vi "add_object.vi"(6 "wait for reply (T)":bool=TRUE, 8 "error in":errorcluster, 9 "object_name":string, 10 "vi_reference":i32) -> (0 "error out":errorcluster, 1 "timed out?":bool, 2 "result":string, 3 "object_id":i32)   [LabVIEW 2025, in "Scripting Server.lvlib"]
doc: "Adds an object to the block diagram or frontpanel of the referenced vi. Get a VI reference from \"New VI\".\nAllowed object names are:\n.NET Container\n.NET Refnum\n2D Picture\n3D Picture\nAbsolute Value\nAccept TLS\nAccess Rights\nActiveX Container\nAdd\nAdd (with error terminals)\nAdd Array Elements\nAdd Entropy\nAdd Private Key To TLS Configuration\nAdd Trusted Certificate To TLS Configuration\nAgitator\nAllSpoll\nAlways Copy\nAnd\nAnd Array Elements\nAppend True/False String\nApplication Refnum\nArray (block diagram constant)\nArray (classic)\nArray (modern)\nArray Interface Control\nArray Max & Min\nArray of Strings to Path\nArray Size\nArray Subset\nArray To Cluster\nArray To Spreadsheet String\nArrayMemInfo\nAssert Structural Type Match\nAssert Structural Type Mismatch\nAtmospheric Tank (classic)\nAtmospheric Tank (modern)\nAutomation Close\nAutomation Open\nAutomation Refnum\nAvogadro Constant (1/mol)\nBase 10 Logarithm Of e\nBin #1\nBin #2\nBitpack to Array\nBluetooth Close Connection\nBluetooth Create Listener\nBluetooth Discover\nBluetooth Network Connection Refnum\nBluetooth Open Connection\nBluetooth Read\nBluetooth Wait On Listener\nBluetooth Write\nBoolean Array To Number\nBoolean To (0,1)\nBuild Array\nBuild Cluster Array\nBuild Map\nBuild Matrix\nBuild Path\nBuild Set\nBuild Waveform\nBundle\nBundle By Name\nByte Array To String\nByte Array To UTF-8 String\nByte Stream File Refnum\nCall By Reference\nCall Chain\nCall Library Function Node\nCall MATLAB Function\nCall Parent Class Method\nCAN Channel (block diagram constant)\nCAN Channel (classic)\nCAN Channel (modern)\nCAN Channel (system)\nCAN Interface (block diagram constant)\nCAN Interface (classic)\nCAN Interface (modern)\nCAN Interface (system)\nCAN Task (block diagram constant)\nCAN Task (classic)\nCAN Task (modern)\nCAN Task (system)\nCancel Button (modern)\nCancel Button (system)\nCancel Notification\nCarriage Return Constant\nCase Structure\nCast Unit Bases\nCheck Valve\nCheckbox (classic)\nCheckBox (modern)\nCheckbox (system)\nClass Specifier Constant\nClassic Color Box\nClassic Color Ramp\nClassic Horizontal Slide Switch\nClassic Vertical Slide\nClear Fixed-Point Overflow Status\nClose File\nClose File (deprecated)\nClose MATLAB Session\nClose Python Session\nClose Reference\nClose TLS Configuration\nClose Variable Connection\nClosure Structure\nCluster (classic)\nCluster (modern)\nCluster Constant\nCluster To Array\nCode Interface Node\nCoerce To Type\nCollection Size\nColor Box Constant\nColor Box Thin Border\nColored Rectangle (broken?)\nCombo Box (classic)\nCombo Box (modern)\nCombo Box (system)\nCombo Box Constant\nComplex Conjugate\nComplex To Polar\nComplex To Re/Im\nCompound Arithmetic\nCompressor\nConcatenate Strings\nConditional Disable Structure\nConstructor Node\nControl & Simulation Loop\nControl Help Window\nControl Online Help\nControl Refnum\nConvert Unit\nConveyer\nCopy\nCopy (deprecated)\nCosecant\nCosine\nCotangent\nCPU Information\nCreate Folder\nCreate Network Stream Endpoint\nCreate Network Stream Reader Endpoint\nCreate Network Stream Writer Endpoint\nCreate Stream\nCreate Unique Network Stream Endpoint\nCreate Unique Network Stream Reader Endpoint\nCreate Unique Network Stream Writer Endpoint\nCreate User Event\nCurrent Processor ID\nCurrent VI's Menubar\nCurrent VI's Path\nDAQmx Analog Trigger Source (block diagram constant)\nDAQmx Analog Trigger Source (classic)\nDAQmx Analog Trigger Source (modern)\nDAQmx Analog Trigger Source (system)\nDAQmx Device Name (block diagram constant)\nDAQmx Device Name (classic)\nDAQmx Device Name (modern)\nDAQmx Device Name (system)\nDAQmx Global Channel (block diagram constant)\nDAQmx Global Channel (classic)\nDAQmx Global Channel (modern)\nDAQmx Global Channel (system)\nDAQmx Physical Channel (block diagram constant)\nDAQmx Physical Channel (classic)\nDAQmx Physical Channel (modern)\nDAQmx Physical Channel (system)\nDAQmx Scale Name (block diagram constant)\nDAQmx Scale Name (classic)\nDAQmx Scale Name (modern)\nDAQmx Scale Name (system)\nDAQmx Switch (block diagram constant)\nDAQmx Switch (classic)\nDAQmx Switch (modern)\nDAQmx Switch (system)\nDAQmx Task Name (block diagram constant)\nDAQmx Task Name (classic)\nDAQmx Task Name (modern)\nDAQmx Task Name (system)\nDAQmx Terminal (block diagram constant)\nDAQmx Terminal (classic)\nDAQmx Terminal (modern)\nDAQmx Terminal (system)\nData Cache Size\nData Log File Refnum\nData Value Reference\nData Value Reference Constant\nDataSocket Close\nDataSocket Open\nDataSocket Read\nDataSocket Refnum\nDataSocket Write\nDate/Time To Seconds\nDecimal Digit?\nDecimal String To Number\nDecimate 1D Array\nDecomposeLockDataValRef\nDecomposeVariant\nDecrement\nDefault Directory\nDelete\nDelete (deprecated)\nDelete Data Value Reference\nDelete From Array\nDelete Menu Items\nDelete Variant Attribute\nDelete Waveform Attribute\nDeny Access\nDequeue Element\nDestroy Stream Endpoint\nDestroy User Event\nDevClear\nDevClearList\nDevice Control/Status\nDevice Refnum\nDiagram Disable Structure\nDial (classic)\nDial (modern)\nDigital Data (classic)\nDigital Data (modern)\nDigital Waveform Graph (classic)\nDigital Waveform Graph (modern)\nDirect Variable Read\nDirect Variable Write\nDivide\nDivide (with error terminals)\nDlg Horiz Scrollbar\nDlg Mac Group Box\nDlg Numeric #1\nDlg Numeric #2\nDlg String\nDlg Vert Scrollbar\nDown Arrow\nDown Bow Valve (flat)\nDown Bow Valve (outline)\nDown Bow Valve (shaded)\nDown Rect Valve (flat)\nDown Rect Valve (outline)\nDown Rect Valve (shaded)\nDown Tee (flat)\nDown Tee (shaded)\nDynamic FPGA Interface Cast\nEased Corner Rectangle\nElement of Set?\nElementary Charge (C)\nEmpty Array?\nEmpty Collection?\nEmpty Path Constant\nEmpty String Constant\nEmpty String/Path?\nEnable Menu Tracking\nEnableLocal\nEnableRemote\nEnd of Line Constant\nEnqueue Element\nEnqueue Element At Opposite End\nEnum (classic)\nEnum (modern)\nEnum (system)\nEnum Constant\nEOF\nEqual To 0?\nEqual?\nError Ring Constant\nEvent Callback Refnum\nEvent Data Node\nEvent Structure\nExchanger\nExclusive Or\nExponential\nExponential (Arg) -1\nExpression Node\nFalse Constant\nFeedback Node\nFieldPoint IO Point (block diagram constant)\nFieldPoint IO Point (classic)\nFieldPoint IO Point (modern)\nFIFO Refnum\nFile Dialog\nFile Dialog (deprecated)\nFile Path Control (classic)\nFile Path Control (modern)\nFile Path Control (system)\nFile Path Indicator (classic)\nFile Path Indicator (modern)\nFile/Directory Info\nFile/Directory Info (deprecated)\nFindLstn\nFindRQS\nFirst Call?\nFixed-Point Overflow?\nFixed-Point to Integer Cast\nFlat Box\nFlat Circle\nFlat Down Triangle\nFlat Frame\nFlat Left Triangle\nFlat Right Triangle\nFlat Round Button\nFlat Rounded Box\nFlat Sequence Structure\nFlat Square Button\nFlat Up Triangle\nFlatten To JSON\nFlatten To String\nFlatten To XML\nFlattened String To Variant\nFloating Point Equal?\nFlush Event Queue\nFlush File\nFlush File (deprecated)\nFlush Queue\nFlush Stream\nFor Loop\nFork\nFormat Date/Time String\nFormat Into File\nFormat Into String\nFormat Value\nFormula Node\nFPGA Refnum to Session\nFract/Exp String To Number\nFramed Color Box (classic)\nFramed Color Box (modern)\nFree Label\nFurnace\nGauge (classic)\nGauge (modern)\nGauge for Simon\nGenerate Front Panel Activity\nGenerate Occurrence\nGenerate User Event\nGenerate User-Defined Trace Event\nGet Control Values by Index\nGet Datalog Position\nGet Date/Time In Seconds\nGet Date/Time String\nGet Drag Drop Data\nGet File Position\nGet File Size\nGet Fixed-Point Components\nGet Help Window Status\nGet Matrix Diagonal\nGet Matrix Elements\nGet Menu Item Info\nGet Menu Selection\nGet Menu Short Cut Info\nGet Notifier Status\nGet Number of Records\nGet Permissions\nGet Queue Status\nGet Submatrix\nGet Type and Creator\nGet Variant Attribute\nGet Volume Info\nGet Waveform Attribute\nGet Waveform Components\nGlobal Variable\nGPIB Clear\nGPIB Initialization\nGPIB Misc\nGPIB Read\nGPIB Serial Poll\nGPIB Status\nGPIB Trigger\nGPIB Wait\nGPIB Write\nGravitational Constant (N m2/kg2)\nGreater Or Equal To 0?\nGreater Or Equal?\nGreater Than 0?\nGreater?\nHandle Peek\nHandle Poke\nHex Digit?\nHexadecimal String To Number\nHopper #1\nHopper #2\nHoriz Line\nHoriz Pipe (flat)\nHoriz Pipe (shaded)\nHorizontal Button Box\nHorizontal Fill Slide (classic)\nHorizontal Fill Slide (modern)\nHorizontal Gradient Oval\nHorizontal Gradient Rectangle\nHorizontal Gradient Rounded Rectangle\nHorizontal Graduated Bar\nHorizontal Pointer Slide (classic)\nHorizontal Pointer Slide (modern)\nHorizontal Pointer Slide (system)\nHorizontal Progress Bar (modern)\nHorizontal Progress Bar (system)\nHorizontal Scrollbar\nHorizontal Slide (classic)\nHorizontal Slide (system)\nHorizontal Smooth Box\nHorizontal Splitter Bar\nHorizontal Splitter Bar (Classic)\nHorizontal Splitter Bar (NXG Style)\nHorizontal Splitter Bar (System)\nHorizontal Switch\nHorizontal Tank\nHorizontal Toggle Switch (classic)\nHorizontal Toggle Switch (modern)\nHyperbolic Cosecant\nHyperbolic Cosine\nHyperbolic Cotangent\nHyperbolic Secant\nHyperbolic Sine\nHyperbolic Tangent\nIMAQ Session\nImplies\nIn Place Element Structure\nIn Range and Coerce\nInclude Fixed-Point Overflow Status\nIncrement\nIndex & Bundle Cluster Array\nIndex Array\nIndex String Array\nInitialize Array\nInline C Node\nInsert Into Array\nInsert Into Map\nInsert Into Set\nInsert Menu Items\nInteger to Fixed-Point Cast\nIntensity Chart (classic)\nIntensity Chart (modern)\nIntensity Graph (classic)\nIntensity Graph (modern)\nInterleave 1D Arrays\nInterpolate 1D Array\nInverse Cosecant\nInverse Cosine\nInverse Cotangent\nInverse Hyperbolic Cosecant\nInverse Hyperbolic Cosine\nInverse Hyperbolic Cotangent\nInverse Hyperbolic Secant\nInverse Hyperbolic Sine\nInverse Hyperbolic Tangent\nInverse Secant\nInverse Sine\nInverse Tangent\nInverse Tangent (2 Input)\nInvoke Node\nIP To String\nIrDA Close Connection\nIrDA Create Listener\nIrDA Discover\nIrDA Network Connection Refnum\nIrDA Open Connection\nIrDA Read\nIrDA Wait On Listener\nIrDA Write\nIsDebuggingActive\nIVI Delete Session\nIVI Logical Name (block diagram constant)\nIVI Logical Name (classic)\nIVI Logical Name (modern)\nIVI New Session\nJoin\nJoin Numbers\nJunction\nKnob (classic)\nKnob (modern)\nLabel (modern)\nLabel (system)\nLabeled Oblong Button\nLabeled Rectangular Button\nLabeled Round Button\nLabeled Square Button\nLabVIEW Object\nLeak Variant Value Reference\nLED Button\nLeft Arrow\nLeft Bow Valve (flat)\nLeft Bow Valve (outline)\nLeft Bow Valve (shaded)\nLeft Down Elbow (flat)\nLeft Down Elbow (shaded)\nLeft Pump (flat)\nLeft Pump (shaded)\nLeft Rect Valve (flat)\nLeft Rect Valve (outline)\nLeft Rect Valve (shaded)\nLeft Tee (flat)\nLeft Tee (shaded)\nLeft Up Elbow (flat)\nLeft Up Elbow (shaded)\nLess Or Equal To 0?\nLess Or Equal?\nLess Than 0?\nLess?\nLexical Class\nLine (chiseled, system)\nLine (chiseled, thick)\nLine (chiseled, thin)\nLine (thick)\nLine (thin)\nLine Feed Constant\nLine with Arrow (thick)\nLine with Arrow (thin)\nList Directory\nList Folder\nListbox (classic)\nListbox (modern)\nListbox (system)\nListbox Symbol Ring Constant\nLoad Certificates Into Memory\nLoad Private Key Into Memory\nLocal Variable\nLock Range\nLogarithm Base 10\nLogarithm Base 2\nLogarithm Base X\nLogical Shift\nLook In Map\nLookup Channel Probe\nLossy Enqueue Element\nLowered Box (thick)\nLowered Rounded Box\nMachine Epsilon\nMake TLS Configuration Immutable\nMakeAddr\nMantissa & Exponent\nMap\nMap Constant\nMatch First String\nMatch Pattern\nMatch True/False String\nMathScript Call By Reference\nMathScript Node\nMATLAB script\nMATLAB Session Refnum\nMatrix Size\nMax & Min\nMenu Refnum\nMenu Ring (classic)\nMenu Ring (modern)\nMenu-Popup Ring\nMerge Errors\nMerge Signals\nMeter (classic)\nMeter (modern)\nMixed Checkbox (system)\nMixed Signal Graph\nMolar Gas Constant (J/(mol K))\nMotion Resource (block diagram constant)\nMotion Resource (classic)\nMotion Resource (modern)\nMotor (flat)\nMotor (shaded)\nMove\nMove (deprecated)\nMulti-Segment Pipe\nMulticolumn Listbox (classic)\nMulticolumn Listbox (modern)\nMulticolumn Listbox (system)\nMultiply\nMultiply (with error terminals)\nMultiply Array Elements\nMultirate Structure\nNatural Logarithm\nNatural Logarithm (Arg +1)\nNatural Logarithm Base\nNatural Logarithm Of 10\nNatural Logarithm Of 2\nNatural Logarithm Of Pi\nNegate\nNegative Infinity\nNew Data Value Reference\nNew Directory\nNew File\nNew TLS Configuration\nNew VI\nNew VI Object\nNot\nNot A Number/Path/Refnum?\nNot A Path Constant\nNot a Refnum Constant\nNot a Shared Variable\nNot And\nNot Equal To 0?\nNot Equal?\nNot Exclusive Or\nNot Or\nNotifier Refnum\nNumber of Cache Levels\nNumber To Boolean Array\nNumber To Decimal String\nNumber To Engineering String\nNumber To Exponential String\nNumber To Fractional String\nNumber To Hexadecimal String\nNumber To Octal String\nNumeric Constant\nNumeric Control (classic)\nNumeric Control (modern)\nNumeric Control (system)\nNumeric Indicator (classic)\nNumeric Indicator (modern)\nObtain Notifier\nObtain Queue\nOccurrence Refnum\nOctal Digit?\nOctal String To Number\nOK Button (modern)\nOK Button (system)\nOld VISA Open\nOLE Variant\nOne Button Dialog\nOpen and Verify Variable Connection\nOpen Application Reference\nOpen Device\nOpen Dynamic Bitfile Reference\nOpen File\nOpen MATLAB Session\nOpen Python Session\nOpen Tank (flat classic)\nOpen Tank (shaded classic)\nOpen Variable Connection\nOpen Variable Connection in Background\nOpen VI Object Reference\nOpen VI Reference\nOpen/Create/Replace Datalog\nOpen/Create/Replace File\nOr\nOr Array Elements\nOval with Shadow\nPackage Matrix\nPassControl\nPath Constant\nPath to Array of Strings\nPath To String\nPath Type\nPi\nPi Divided By 2\nPi Multiplied By 2\nPick Line\nPict Ring (classic)\nPict Ring (modern)\nPict Ring (system)\nPixMap\nPixMap (warning: dangerous)\nPlanck's Constant (J/Hz)\nPlatform Flat Square Button\nPlug-In Control\nPolar To Complex\nPolar To Re/Im\nPositive Infinity\nPower Of 10\nPower Of 2\nPower Of X\nPPoll\nPPollConfig\nPPollUnconfig\nPreallocated Read from Binary File\nPreserve Run-Time Class\nPressure Tank (flat)\nPressure Tank (shaded)\nPreview Queue Element\nPrintable?\nProperty Node\nPulldown Menu Ring\nPush Button\nPython Node\nPython Session Refnum\nQueue Refnum\nQuit LabVIEW\nQuotient & Remainder\nRace Structure\nRadio Button (system)\nRadio Buttons (classic)\nRadio Buttons (modern)\nRadio Buttons (system)\nRaised Box (classic)\nRaised Box (modern)\nRaised Circle\nRaised Down Triangle\nRaised Frame\nRaised Left Triangle\nRaised Right Triangle\nRaised Rounded Box\nRaised Up Triangle\nRandom Number (0-1)\nRcvRespMsg\nRe-accept TLS\nRe/Im To Complex\nRe/Im To Polar\nRead Datalog\nRead Device\nRead File\nRead from Binary File\nRead from Text File\nRead Map Max & Min Keys\nRead Multiple Elements from Stream\nRead Set Max & Min\nRead Single Element from Stream\nRead Variable\nRead Variable with Timeout\nReadStatus\nReceive\nReceiveSetup\nRecessed Box\nRecessed Circle\nRecessed Down Triangle\nRecessed Frame (modern)\nRecessed Frame (system)\nRecessed Left Triangle\nRecessed Menu Ring\nRecessed Right Triangle\nRecessed Rounded Box\nRecessed Up Triangle\nReciprocal\nReciprocal Of e\nReciprocal Of Pi\nRecomposeUnlockDataValRef (warning: dangerous)\nRecomposeVariant (warning: dangerous)\nRectangular Stop Button\nRefnum to Path\nRefnum to Session\nRegion\nRegister Event Callback\nRegister For Events\nRegister Session\nRelease Notifier\nRelease Queue\nRemove Fixed-Point Overflow Status\nRemove From Map\nRemove From Set\nReplace Array Subset\nReplace Substring\nRequest Deallocation\nResetSys\nReshape Array\nResize Matrix\nResource Index\nReverse 1D Array\nReverse String\nRight Arrow\nRight Bow Valve (flat)\nRight Bow Valve (outline)\nRight Bow Valve (shaded)\nRight Down Elbow (flat)\nRight Down Elbow (shaded)\nRight Pump (flat)\nRight Pump (shaded)\nRight Rect Valve (flat)\nRight Rect Valve (outline)\nRight Rect Valve (shaded)\nRight Tee (flat)\nRight Tee (shaded)\nRight Up Elbow (flat)\nRight Up Elbow (shaded)\nRocker\nRotary Feeder\nRotate\nRotate 1D Array\nRotate Left With Carry\nRotate Right With Carry\nRotate String\nRound Button\nRound LED (classic)\nRound LED (modern)\nRound Light\nRound Push Button\nRound Push Button (profile)\nRound Radio Button\nRound Stop Button\nRound To Nearest\nRound Toward +Infinity\nRound Toward -Infinity\nRounded Rectangle with Shadow\nRT FIFO Create\nRT FIFO Delete\nRT FIFO Read\nRT FIFO Write\nRydberg Constant (1/m)\nScale By Power Of 2\nScan From File\nScan From String\nScan String For Tokens\nScan Value\nScanned Variable Read\nScanned Variable Write\nSearch 1D Array\nSearch and Replace String\nSearch Variable Container\nSearch/Split String\nSecant\nSeconds To Date/Time\nSeek\nSelect\nSend\nSend Notification\nSendCmds\nSendDataBytes\nSendIFC\nSendList\nSendLLO\nSendSetup\nSession to Refnum\nSet\nSet Constant\nSet Control Values by Index\nSet Datalog Position\nSet File Position\nSet File Size\nSet Matrix Diagonal\nSet Matrix Elements\nSet Menu Item Info\nSet Number of Records\nSet Occurrence\nSet Permissions\nSet Submatrix\nSet Type and Creator\nSet Variant Attribute\nSet Waveform Attribute\nSetRWLS\nSetTimeOut\nShared Variable\nShared Variable Constant\nShared Variable Control (classic)\nShared Variable Control (modern)\nShared Variable to String\nSign\nSimple Horizontal Slide\nSimple Numeric\nSimple String\nSimple Vertical Slide\nSinc\nSine\nSine & Cosine\nSize Handle\nSlide Switch\nSmoothed Oval\nSmoothed Rounded Rectangle\nSort 1D Array\nSort Array of String\nSpeed Of Light In Vacuum (m/sec)\nSpin Control (system)\nSplit 1D Array\nSplit Button\nSplit Number\nSplit Signals\nSpreadsheet String To Array\nSquare\nSquare Button\nSquare LED (classic)\nSquare LED (modern)\nSquare Light\nSquare Push Button\nSquare Push Button (profile)\nSquare Radio Button\nSquare Root\nStacked Sequence Structure\nStart TLS\nState\nState Diagram\nStatic VI Reference\nStop\nStop Button\nString Constant\nString Control (classic)\nString Control (modern)\nString Control (system)\nString Indicator (classic)\nString Indicator (modern)\nString Length\nString Subset\nString To Byte Array\nString To IP\nString To Path\nString to Shared Variable\nStrip Path\nSubPanel\nSubPanel (Classic)\nSubPanel (NXG Style)\nSubPanel (System)\nSubtract\nSubtract (with error terminals)\nSwap Bytes\nSwap Values\nSwap Vector Element\nSwap Words\nTab Constant\nTab Control (classic)\nTab Control (modern)\nTab Control (NXG Style)\nTab Control (system)\nTable (classic)\nTable (modern)\nTable (system)\nTag Attribute Ring\nTangent\nTank (classic)\nTank (modern)\nTarget Structure\nTCP Close Connection\nTCP Create Listener\nTCP Flattened Read\nTCP Flattened Write\nTCP Flex Read\nTCP Flex Write\nTCP Network Connection Refnum\nTCP Open Connection\nTCP Read\nTCP Wait On Listener\nTCP Write\nTDMS Advanced Asynchronous Read (Data Ref)\nTDMS Advanced Asynchronous Write (Data Ref)\nTDMS Close\nTDMS Configure Asynchronous Reads (Data Ref)\nTDMS Configure Asynchronous Writes (Data Ref)\nTDMS Defragment\nTDMS Delete Data\nTDMS File\nTDMS Flush\nTDMS Get Asynchronous Read Status (Data Ref)\nTDMS Get Asynchronous Write Status (Data Ref)\nTDMS Get Properties\nTDMS In Memory Close\nTDMS In Memory Open\nTDMS In Memory Read Bytes\nTDMS List Contents\nTDMS Open\nTDMS Read\nTDMS Refnum To File ID\nTDMS Set Properties\nTDMS Write\nTDMS Write IP\nTemporary Directory\nTestSRQ\nTestSys\nText & Pict Ring (classic)\nText & Pict Ring (modern)\nText Button\nText Ring (block diagram constant)\nText Ring (classic)\nText Ring (modern)\nText Ring (system)\nText to UTF-8\nThermometer (classic)\nThermometer (modern)\nThreshold 1D Array\nTick Count (ms)\nTime Stamp (block diagram constant)\nTime Stamp Control (classic)\nTime Stamp Control (modern)\nTime Stamp Control (system)\nTime Stamp Indicator (classic)\nTime Stamp Indicator (modern)\nTimed Loop\nTimed Sequence\nTLS configuration\nTLS Connection?\nTo Byte Integer\nTo Double Precision Complex\nTo Double Precision Float\nTo Extended Precision Complex\nTo Extended Precision Float\nTo Fixed-Point\nTo Long Integer\nTo Lower Case\nTo More Generic Class\nTo More Specific Class\nTo OLE Variant\nTo Probe String\nTo Quad Integer\nTo Single Precision Complex\nTo Single Precision Float\nTo Time Stamp\nTo Unsigned Byte Integer\nTo Unsigned Long Integer\nTo Unsigned Quad Integer\nTo Unsigned Word Integer\nTo Upper Case\nTo Variant\nTo Word Integer\nTraditional DAQ Channel (block diagram constant)\nTraditional DAQ Channel (classic)\nTraditional DAQ Channel (modern)\nTranspose 1D Array\nTranspose 2D Array\nTranspose Matrix\nTree (classic)\nTree (modern)\nTree (system)\nTrigger\nTriggerList\nTwo Button Dialog\nType and Creator\nType Cast\nType Error\nType Must Be Array\nType Must Be Cluster\nType Of\nType Specialization Structure\nUDP Close\nUDP Multicast Open\nUDP Network Connection Refnum\nUDP Open\nUDP Read\nUDP Write\nUnbitpack from Array\nUnbundle\nUnbundle By Name\nUnflatten From JSON\nUnflatten From String\nUnflatten From XML\nUnleak Variant Value Reference\nUnpackage Matrix\nUnregister For Events\nUnregister Session\nUp Arrow\nUp Bow Valve (flat)\nUp Bow Valve (outline)\nUp Bow Valve (shaded)\nUp Rect Valve (flat)\nUp Rect Valve (outline)\nUp Rect Valve (shaded)\nUp Tee (flat)\nUp Tee (shaded)\nUser Defined Refnum\nUser Defined Refnum Tag (block diagram constant)\nUser Defined Refnum Tag (classic)\nUser Defined Refnum Tag (modern)\nUser Defined Refnum Tag Flatten (classic)\nUser Defined Refnum Tag Flatten (modern)\nUser Defined Tag (block diagram constant)\nUser Defined Tag (classic)\nUser Defined Tag (modern)\nUser Item\nUTF-8 String To Byte Array\nUTF-8 to Text\nVariable Class Specifier Constant\nVariable Name Constant\nVariant\nVariant To Data\nVariant To Flattened String\nVert Line\nVert Pipe (flat)\nVert Pipe (shaded)\nVert Rocker\nVertical Fill Slide (classic)\nVertical Fill Slide (modern)\nVertical Gradient Oval\nVertical Gradient Rectangle\nVertical Gradient Rounded Rectangle\nVertical Graduated Bar\nVertical Pointer Slide (classic)\nVertical Pointer Slide (modern)\nVertical Pointer Slide (system)\nVertical Progress Bar (modern)\nVertical Progress Bar (system)\nVertical Scrollbar\nVertical Slide (system)\nVertical Slide Switch (classic)\nVertical Slide Switch (modern)\nVertical Smooth Box\nVertical Splitter Bar\nVertical Splitter Bar (Classic)\nVertical Splitter Bar (NXG Style)\nVertical Splitter Bar (System)\nVertical Switch\nVertical Toggle Switch (classic)\nVertical Toggle Switch (modern)\nVI Library\nVI Refnum\nVI Server Reference\nVISA Assert Interrupt Signal\nVISA Assert Trigger\nVISA Assert Utility Signal\nVISA Clear\nVISA Close\nVISA Disable Event\nVISA Discard Events\nVISA Enable Event\nVISA Find Resource\nVISA Flush I/O Buffer\nVISA GPIB Command\nVISA GPIB Control ATN\nVISA GPIB Control REN\nVISA GPIB Pass Control\nVISA GPIB Send IFC\nVISA In 16\nVISA In 32\nVISA In 64\nVISA In 8\nVISA Lock\nVISA Map Address\nVISA Map Trigger\nVISA Memory Allocation\nVISA Memory Allocation Ex\nVISA Memory Free\nVISA Move\nVISA Move In 16\nVISA Move In 32\nVISA Move In 64\nVISA Move In 8\nVISA Move Out 16\nVISA Move Out 32\nVISA Move Out 64\nVISA Move Out 8\nVISA Open\nVISA Out 16\nVISA Out 32\nVISA Out 64\nVISA Out 8\nVISA Peek 16\nVISA Peek 32\nVISA Peek 64\nVISA Peek 8\nVISA Poke 16\nVISA Poke 32\nVISA Poke 64\nVISA Poke 8\nVISA Read\nVISA Read STB\nVISA Read To File\nVISA Refnum to Session\nVISA Resource Name\nVISA resource name (classic)\nVISA resource name (modern)\nVISA Set I/O Buffer Size\nVISA Status Description\nVISA Unlock\nVISA Unmap Address\nVISA Unmap Trigger\nVISA USB Control In\nVISA USB Control Out\nVISA VXI Cmd or Query\nVISA Wait on Event\nVISA Write\nVISA Write From File\nVolume Info\nWait (ms)\nWait For Activity\nWait For Front Panel Activity\nWait for GPIB RQS\nWait on Notification\nWait on Notification from Multiple\nWait on Notification from Multiple with Notifier History\nWait on Notification with Notifier History\nWait on Occurrence\nWait Until Next ms Multiple\nWaitSRQ\nWaveform Chart\nWaveform Chart (classic)\nWaveform Chart (modern)\nWaveform Graph (classic)\nWaveform Graph (modern)\nWhile Loop #1\nWhile Loop #2\nWhite Space?\nWrite Datalog\nWrite Device\nWrite File\nWrite Multiple Elements to Stream\nWrite Single Element to Stream\nWrite to Binary File\nWrite to Text File\nWrite Variable\nWrite Variable with Timeout\nXY Graph (classic)\nXY Graph (modern)\nY-th Root of X"
uses:
  Scripting Server.lvlib
  Add Object Argument--cluster.ctl
  Add Object (Reply Payload)--cluster.ctl
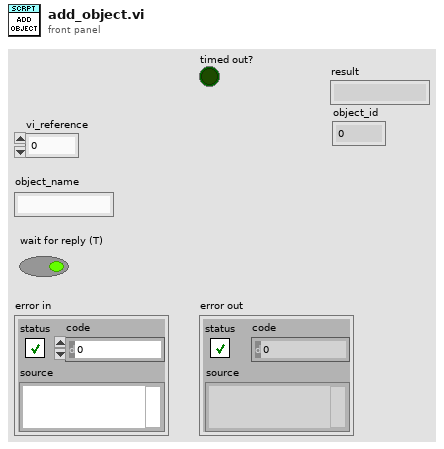
[diagram p1: front panel]
types:
  T1 = typedef "Scripting Server.lvlib/Add Object Argument--cluster.ctl" = cluster{"VI Reference":i32, "Object Name":string, "Wait Notifier":refnum<notifier>, "wait for reply":bool}
  T2 = typedef "Scripting Server.lvlib/Request Events--cluster.ctl" = cluster{"Stop Module":refnum<user-event>, "Show Panel":refnum<user-event>, "Hide Panel":refnum<user-event>, "Get Module Execution Status":refnum<user-event>, "Show Diagram":refnum<user-event>, "New VI":refnum<user-event>, "Add Object":refnum<user-event>, "Connect Objects":refnum<user-event>, "Get Object Terminals":refnum<user-event>, "get vi error list":refnum<user-event>, "Cleanup VI":refnum<user-event>, "create_control":refnum<user-event>, "Run VI":refnum<user-event>}
  T3 = typedef "Scripting Server.lvlib/Add Object (Reply Payload)--cluster.ctl" = cluster{"error":errorcluster, "Object ID":i32, "Result":string}
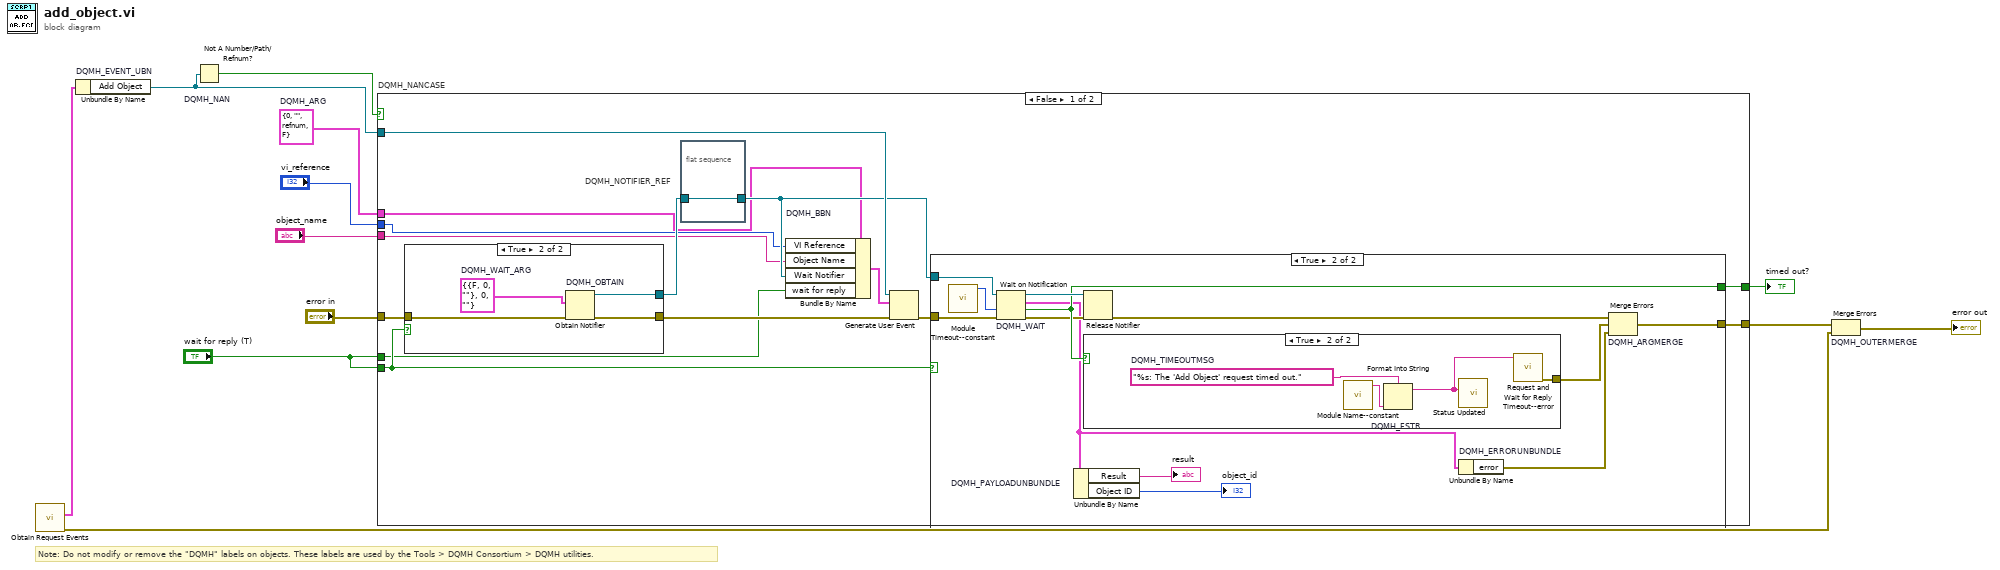
[diagram p0: block diagram]
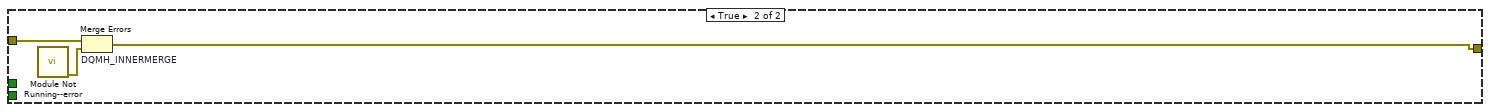
[diagram p5: hidden frame]
diagram:
  w6 = T1 {"VI Reference"=0, "Object Name"="", "Wait Notifier"=refnum, "wait for reply"=FALSE}  # DQMH_ARG
  # "Note: Do not modify or remove the \"DQMH\" labels on objects. These labels are used by the Tools > DQMH Consortium > DQMH utilities."
  n1 = call "Obtain Request Events.vi"() -> ("error out"=w2:errorcluster, "Scripting Server Request Events"=w1:T2)  [unwired: 10 in]
  n2 = Unbundle By Name "DQMH_EVENT_UBN"(w1) -> ("Add Object"=w7:refnum<user-event>)
  n3 = Not A Number/Path/Refnum? "DQMH_NAN"(number/path/refnum=w7) -> (NaN/Path/Refnum?=w8:bool)
  n4 = case "DQMH_NANCASE" shown="False" w8 {
    tunnel: "error in" -> [w26 w53]
    tunnel: w7 -> [w24 _]
    tunnel: [w21 w52] -> w9
    tunnel: [w22 _] -> w11
    tunnel: "wait for reply (T)" -> [w19 _]
    tunnel: w6 -> [w16 _]
    tunnel: "vi_reference" -> [w15 _]
    tunnel: "object_name" -> [w14 _]
    tunnel: "wait for reply (T)" -> [w13 _]
    frame False {
      n5 = case shown="True" w19 {
        tunnel: w26 -> [w46 w50]
        tunnel: [w46 w49] -> w23
        tunnel: [_ w47] -> w18
        frame False {
        }
        frame True {
          w48 = T3 {"error"={"status"=FALSE, "code"=0, "source"=""}, "Object ID"=0, "Result"=""}  # DQMH_WAIT_ARG
          n6 = Obtain Notifier "DQMH_OBTAIN"(notification data type=w48, error in (no error)=w50) -> (notifier out=w47:refnum<notifier>, error out=w49:errorcluster)  [unwired: 2 in, 1 out]
        }
      }
      n7 = flat-sequence "DQMH_NOTIFIER_REF" {
        tunnel: w18 -> [w27]
        tunnel: [w27] -> w17
        frame #0 {
        }
      }
      n8 = Bundle By Name "DQMH_BBN"(cluster=w16, "VI Reference"=w15, "Object Name"=w14, "Wait Notifier"=w17, "wait for reply"=w13) -> (w20:T1)
      n9 = Generate User Event(user event=w24, event data cluster=w20, error in=w23) -> (error out=w25:errorcluster)  [unwired: 1 in, 1 out]
      n10 = case shown="True" w19 {
        tunnel: w25 -> [w28 w41]
        tunnel: w17 -> [_ w40]
        tunnel: [_ w38] -> w22
        tunnel: [w28 w37] -> w21
        frame False {
        }
        frame True {
          n11 = call "Module Timeout--constant.vi"() -> ("Module Timeout"=w31:i32)  [unwired: 11 in]
          n12 = Wait on Notification "DQMH_WAIT"(notifier=w40, timeout in ms (-1)=w31, error in (no error)=w41) -> (notifier out=w39:refnum<notifier>, notification=w32:T3, timed out?=w38:bool, error out=w36:errorcluster)  [unwired: 1 in]
          n13 = Unbundle By Name "DQMH_PAYLOADUNBUNDLE"(w32) -> ("Result"=→"result":string, "Object ID"=→"object_id":i32)
          n14 = Release Notifier(notifier=w39, error in (no error)=w36) -> (error out=w35:errorcluster)  [unwired: 1 in, 2 out]
          n15 = case shown="True" w38 {
            tunnel: [_ w43] -> w33
            frame False {
            }
            frame True {
              w45 = "%s: The 'Add Object' request timed out."  # DQMH_TIMEOUTMSG
              n16 = call "Module Name--constant.vi"() -> ("Module Name"=w42:string)  [unwired: 11 in]
              n17 = Format Into String "DQMH_FSTR"(format string=w45, w42) -> (resulting string=w44:string)  [unwired: 2 in, 1 out]
              n18 = call "Status Updated.vi"("Status"=w44) -> ()  [unwired: 10 in, 1 out]
              n19 = call "Request and Wait for Reply Timeout--error.vi"("Error Message"=w44) -> ("error out"=w43:errorcluster)  [unwired: 10 in]
            }
          }
          n20 = Unbundle By Name "DQMH_ERRORUNBUNDLE"(w32) -> ("error"=w34:errorcluster)
          n21 = Merge Errors "DQMH_ARGMERGE"(w35, w33, w34) -> (w37:errorcluster)
        }
      }
    }
    frame True {
      n22 = call "Module Not Running--error.vi"() -> ("error out"=w51:errorcluster)  [unwired: 11 in]
      n23 = Merge Errors "DQMH_INNERMERGE"(w53, w51) -> (w52:errorcluster)
    }
  }
  "timed out?" <- w11
  n24 = Merge Errors "DQMH_OUTERMERGE"(w9, w2) -> (→"error out":errorcluster)
